vi "S2C_UTILITY_Proc_Commands.vi"(8 "Error In":errorcluster, 10 "Settings":T1, 11 "Q-Ref":refnum<queue>) -> (0 "Error Out":errorcluster, 2 "Stop?":bool, 3 "Response":variant)   [LabVIEW 2015]
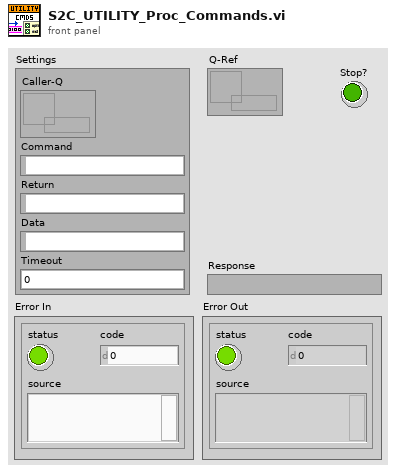
[diagram p1: front panel]
types:
  T1 = cluster{"Caller-Q":refnum<queue>, "Command":string, "Return":string, "Data":variant, "Timeout":dbl}
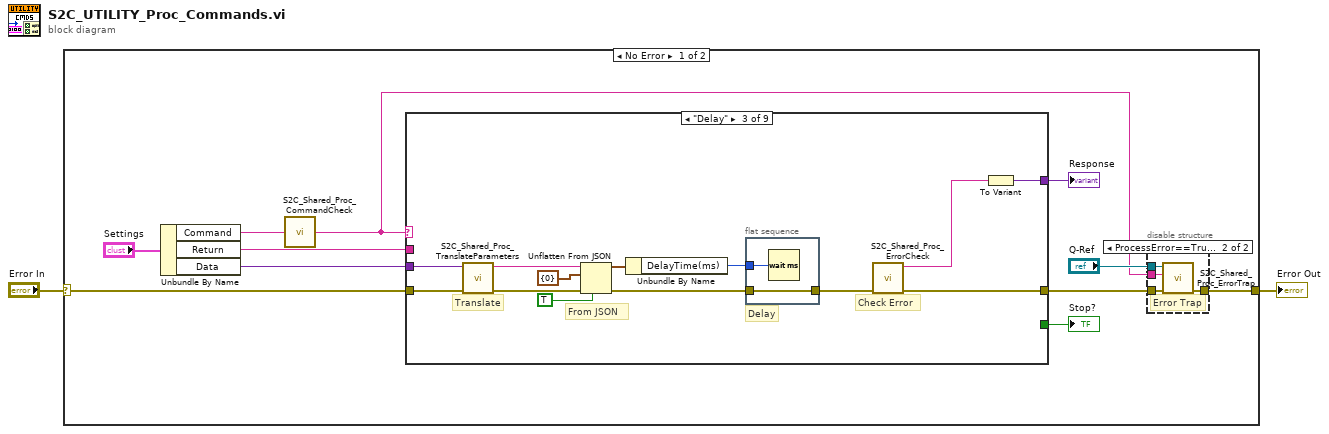
[diagram p0: block diagram]
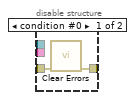
[diagram p2: hidden frame]
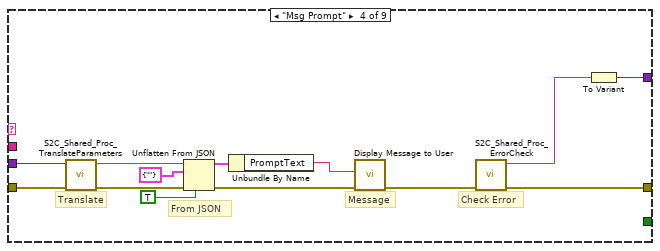
[diagram p5: hidden frame]
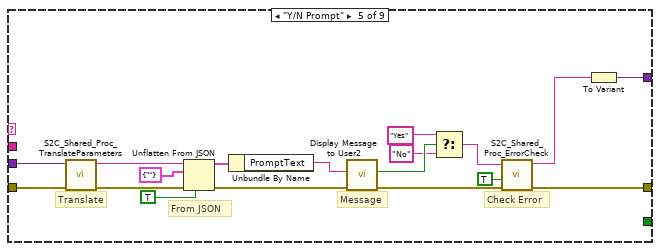
[diagram p6: hidden frame]
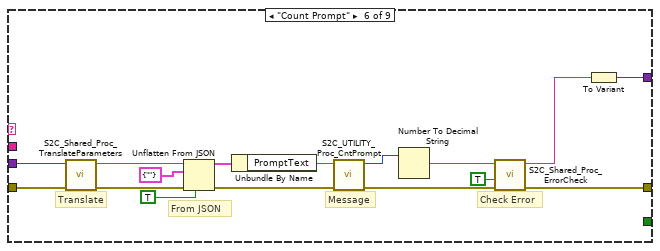
[diagram p7: hidden frame]
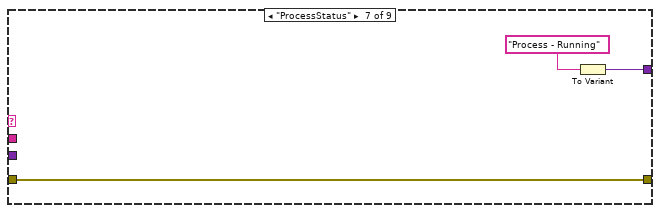
[diagram p8: hidden frame]
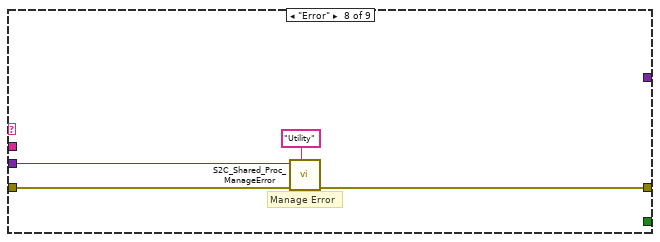
[diagram p9: hidden frame]
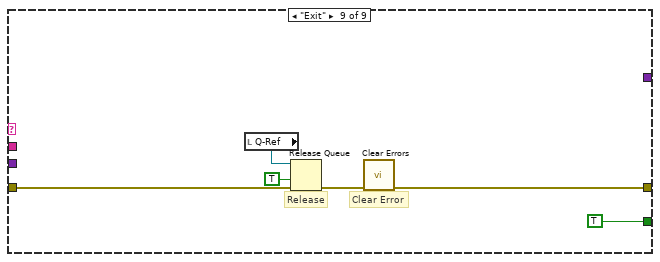
[diagram p10: hidden frame]
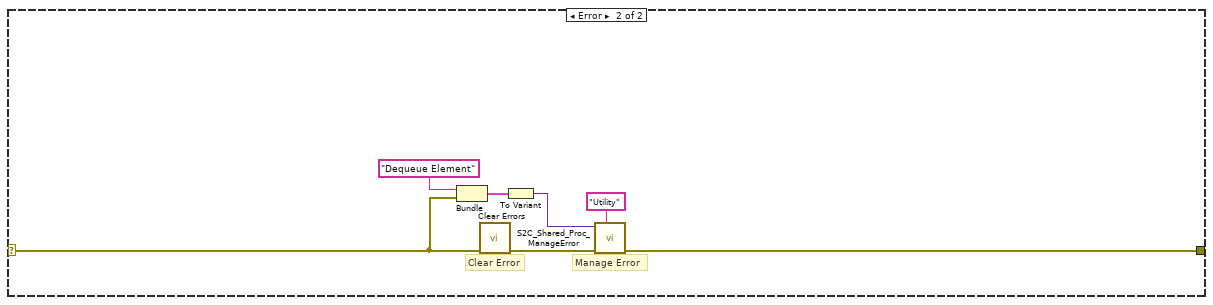
[diagram p11: hidden frame]
diagram:
  n1 = case shown="No Error" "Error In" {
    selector: "Error In" -> [w12 w100]
    tunnel: [w5 w102] -> w1
    frame No Error {
      n2 = Unbundle By Name("Settings") -> ("Command"=w4:string, "Return"=w8:string, "Data"=w13:variant)
      n3 = call "S2C_Shared_Proc_CommandCheck.vi"("Cmd In"=w4) -> ("Cmd Out"=w3:string)  [unwired: 13 in, 1 out]
      n4 = case shown="\"Delay\"" w3 {
        tunnel: w12 -> [w20 w21 w34 w49 w67 w83 w84 w89 w91]
        tunnel: w13 -> [_ _ w33 w48 w66 w82 _ w87 _]
        tunnel: [w20 w21 w24 w41 w59 w75 w84 w88 w92] -> w6
        tunnel: [_ _ w26 w42 w60 w76 w85 _ _] -> w10
        tunnel: [_ _ _ _ _ _ _ _ TRUE] -> w9
        tunnel: w8 -> [_ _ _ _ _ _ _ _ _]
        frame "Other", Default {
        }
        frame "Init" {
        }
        frame "Delay" {
          # "Check Error"
          # "Delay"
          # "From JSON"
          # "Translate"
          n5 = call "S2C_Shared_Proc_TranslateParameters.vi"("Error In"=w34, "Data"=w33) -> ("Error Out"=w31:errorcluster, "JSON Cluster"=w30:string)  [unwired: 8 in]
          n6 = Unflatten From JSON(JSON string=w30, type and defaults=cluster{"DelayTime(ms)":u32} {"DelayTime(ms)"=0}, default null elements? (F)=TRUE, error in (no error)=w31) -> (value=w28:cluster{"DelayTime(ms)":u32}, error out=w22:errorcluster)  [unwired: 3 in]
          n7 = Unbundle By Name(w28) -> ("DelayTime(ms)"=w27:u32)
          n8 = flat-sequence {
            tunnel: w22 -> [w35]
            tunnel: w27 -> [w36]
            tunnel: [w35] -> w25
            frame #0 {
              n9 = Wait (ms)(milliseconds to wait=w36) -> ()  [unwired: 1 out]
            }
          }
          n10 = call "S2C_Shared_Proc_ErrorCheck.vi"("Error In"=w25) -> ("Error Out"=w24:errorcluster, "Status"=w23:string)  [unwired: 9 in]
          n11 = To Variant(anything=w23) -> (Variant=w26:variant)
        }
        frame "Msg Prompt" {
          # "Check Error"
          # "Message"
          # "From JSON"
          # "Translate"
          n12 = call "S2C_Shared_Proc_TranslateParameters.vi"("Error In"=w49, "Data"=w48) -> ("Error Out"=w46:errorcluster, "JSON Cluster"=w45:string)  [unwired: 8 in]
          n13 = Unflatten From JSON(JSON string=w45, type and defaults=cluster{"PromptText":string} {"PromptText"=""}, default null elements? (F)=TRUE, error in (no error)=w46) -> (value=w43:cluster{"PromptText":string}, error out=w39:errorcluster)  [unwired: 3 in]
          n14 = Unbundle By Name(w43) -> ("PromptText"=w38:string)
          n15 = call "Display Message to User"("error in (no error)"=w39, "Message"=w38) -> ("error out"=w37:errorcluster)  [unwired: 8 in, 1 out]
          n16 = call "S2C_Shared_Proc_ErrorCheck.vi"("Error In"=w37) -> ("Error Out"=w41:errorcluster, "Status"=w40:string)  [unwired: 9 in]
          n17 = To Variant(anything=w40) -> (Variant=w42:variant)
        }
        frame "Y/N Prompt" {
          # "Check Error"
          # "Message"
          # "From JSON"
          # "Translate"
          n18 = call "S2C_Shared_Proc_TranslateParameters.vi"("Error In"=w67, "Data"=w66) -> ("Error Out"=w64:errorcluster, "JSON Cluster"=w63:string)  [unwired: 8 in]
          n19 = Unflatten From JSON(JSON string=w63, type and defaults=cluster{"PromptText":string} {"PromptText"=""}, default null elements? (F)=TRUE, error in (no error)=w64) -> (value=w61:cluster{"PromptText":string}, error out=w57:errorcluster)  [unwired: 3 in]
          n20 = Unbundle By Name(w61) -> ("PromptText"=w56:string)
          n21 = call "Display Message to User2"("error in (no error)"=w57, "Message"=w56) -> ("error out"=w55:errorcluster, "Yes"=w54:bool)  [unwired: 8 in]
          n22 = Select(t="Yes", s=w54, f="No") -> (s? t:f=w51:string)
          n23 = call "S2C_Shared_Proc_ErrorCheck.vi"("Error In"=w55, "ExpReply?"=TRUE, "Reply Text"=w51) -> ("Error Out"=w59:errorcluster, "Status"=w58:string)  [unwired: 7 in]
          n24 = To Variant(anything=w58) -> (Variant=w60:variant)
        }
        frame "Count Prompt" {
          # "Check Error"
          # "Message"
          # "From JSON"
          # "Translate"
          n25 = call "S2C_Shared_Proc_TranslateParameters.vi"("Error In"=w83, "Data"=w82) -> ("Error Out"=w80:errorcluster, "JSON Cluster"=w79:string)  [unwired: 8 in]
          n26 = Unflatten From JSON(JSON string=w79, type and defaults=cluster{"PromptText":string} {"PromptText"=""}, default null elements? (F)=TRUE, error in (no error)=w80) -> (value=w77:cluster{"PromptText":string}, error out=w72:errorcluster)  [unwired: 3 in]
          n27 = Unbundle By Name(w77) -> ("PromptText"=w70:string)
          n28 = call "S2C_UTILITY_Proc_CntPrompt.vi"("Error In"=w72, "Message"=w70) -> ("Error Out"=w71:errorcluster, "Cnt"=w69:i32)  [unwired: 8 in]
          n29 = Number To Decimal String(number=w69) -> (decimal integer string=w68:string)  [unwired: 1 in]
          n30 = call "S2C_Shared_Proc_ErrorCheck.vi"("Error In"=w71, "ExpReply?"=TRUE, "Reply Text"=w68) -> ("Error Out"=w75:errorcluster, "Status"=w74:string)  [unwired: 7 in]
          n31 = To Variant(anything=w74) -> (Variant=w76:variant)
        }
        frame "ProcessStatus" {
          n32 = To Variant(anything="Process - Running") -> (Variant=w85:variant)
        }
        frame "Error" {
          # "Manage Error"
          n33 = call "S2C_Shared_Proc_ManageError.vi"("Process"="Utility", "Error In"=w89, "Data"=w87) -> ("Error Out"=w88:errorcluster)  [unwired: 8 in]
        }
        frame "Exit" {
          # "Clear Error"
          # "Release"
          n34 = local read "Q-Ref"() -> (w94:refnum<queue>)
          n35 = Release Queue(queue=w94, force destroy? (F)=TRUE, error in (no error)=w91) -> (error out=w95:errorcluster)  [unwired: 2 out]
          n36 = call <vilib>:"Clear Errors.vi"("error in (no error)"=w95) -> ("error out"=w92:errorcluster)  [unwired: 5 in, 1 out]
        }
      }
      "Response" <- w10
      "Stop?" <- w9
      n37 = disable-structure shown="ProcessError==True" {
        disable-tunnel: w6 -> [w15 w19]
        disable-tunnel: [w14 w18] -> w5
        disable-tunnel: w3 -> [_ w17]
        disable-tunnel: "Q-Ref" -> [_ w16]
        frame condition #0 {
          n38 = call <vilib>:"Clear Errors.vi"("error in (no error)"=w15) -> ("error out"=w14:errorcluster)  [unwired: 5 in, 1 out]
        }
        frame condition #1 (active) {
          # "Error Trap"
          n39 = call "S2C_Shared_Proc_ErrorTrap.vi"("Error In"=w19, "Command"=w17, "Q-Ref"=w16) -> ("Error Out"=w18:errorcluster)  [unwired: 8 in]
        }
      }
    }
    frame Error {
      # "Clear Error"
      # "Manage Error"
      n40 = Bundle("Dequeue Element", "error IO"=w100) -> (w101:cluster{string, "error IO":errorcluster})  [unwired: 1 in]
      n41 = call <vilib>:"Clear Errors.vi"("error in (no error)"=w100) -> ("error out"=w97:errorcluster)  [unwired: 5 in, 1 out]
      n42 = To Variant(anything=w101) -> (Variant=w98:variant)
      n43 = call "S2C_Shared_Proc_ManageError.vi"("Process"="Utility", "Error In"=w97, "Data"=w98) -> ("Error Out"=w102:errorcluster)  [unwired: 8 in]
    }
  }
  "Error Out" <- w1
